vi "GetLastError.vi"() -> (3 "function return":string)   [LabVIEW 2015, in "IRB.lvlib"]
doc: "const char* IRB_EXPORT irb_get_last_error(void);"
uses:
  IRB.lvlib
  IRB.dll
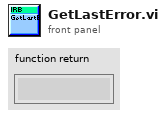
[diagram p1: front panel]
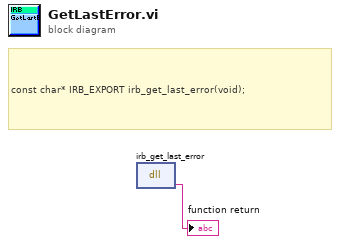
[diagram p0: block diagram]
diagram:
  # "const char* IRB_EXPORT irb_get_last_error(void);"
  n1 = dll-call lib="C:/LabView/IRB/x86_32/IRB.*" fn="irb_get_last_error"() -> ("return type"=→"function return":string)  [unwired: 3 in, 2 out]
